vi "OP600ZP_CLUSTER_SOFTS.vi"(10 "MESURES":T1, 11 "EmptyTab":string[][](array[string])) -> (4 "Tab1":string[][](array[string]), 6 "PASS/FAIL":bool[](array[boolean]))   [LabVIEW 2020]
uses:
  VG/PackType.vi
  VG/IS30%.vi
  OP600ZP_VGConf.vi
panel:
  out "VG IS30% ?":bool
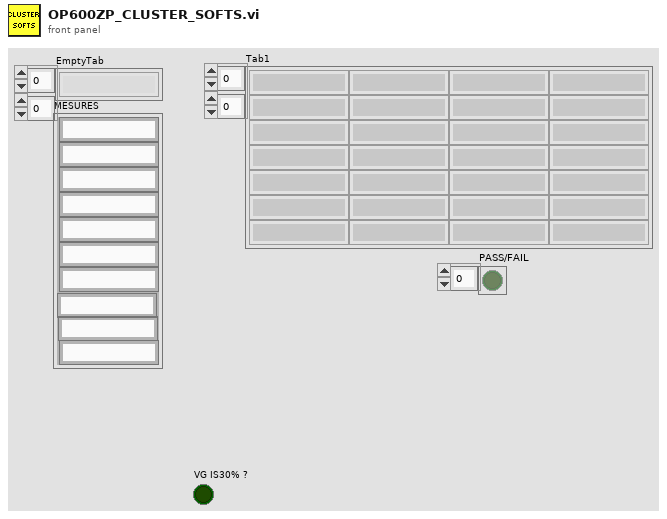
[diagram p1: front panel]
types:
  T1 = cluster{string, string, string, string, string, string, string, string, string, string}
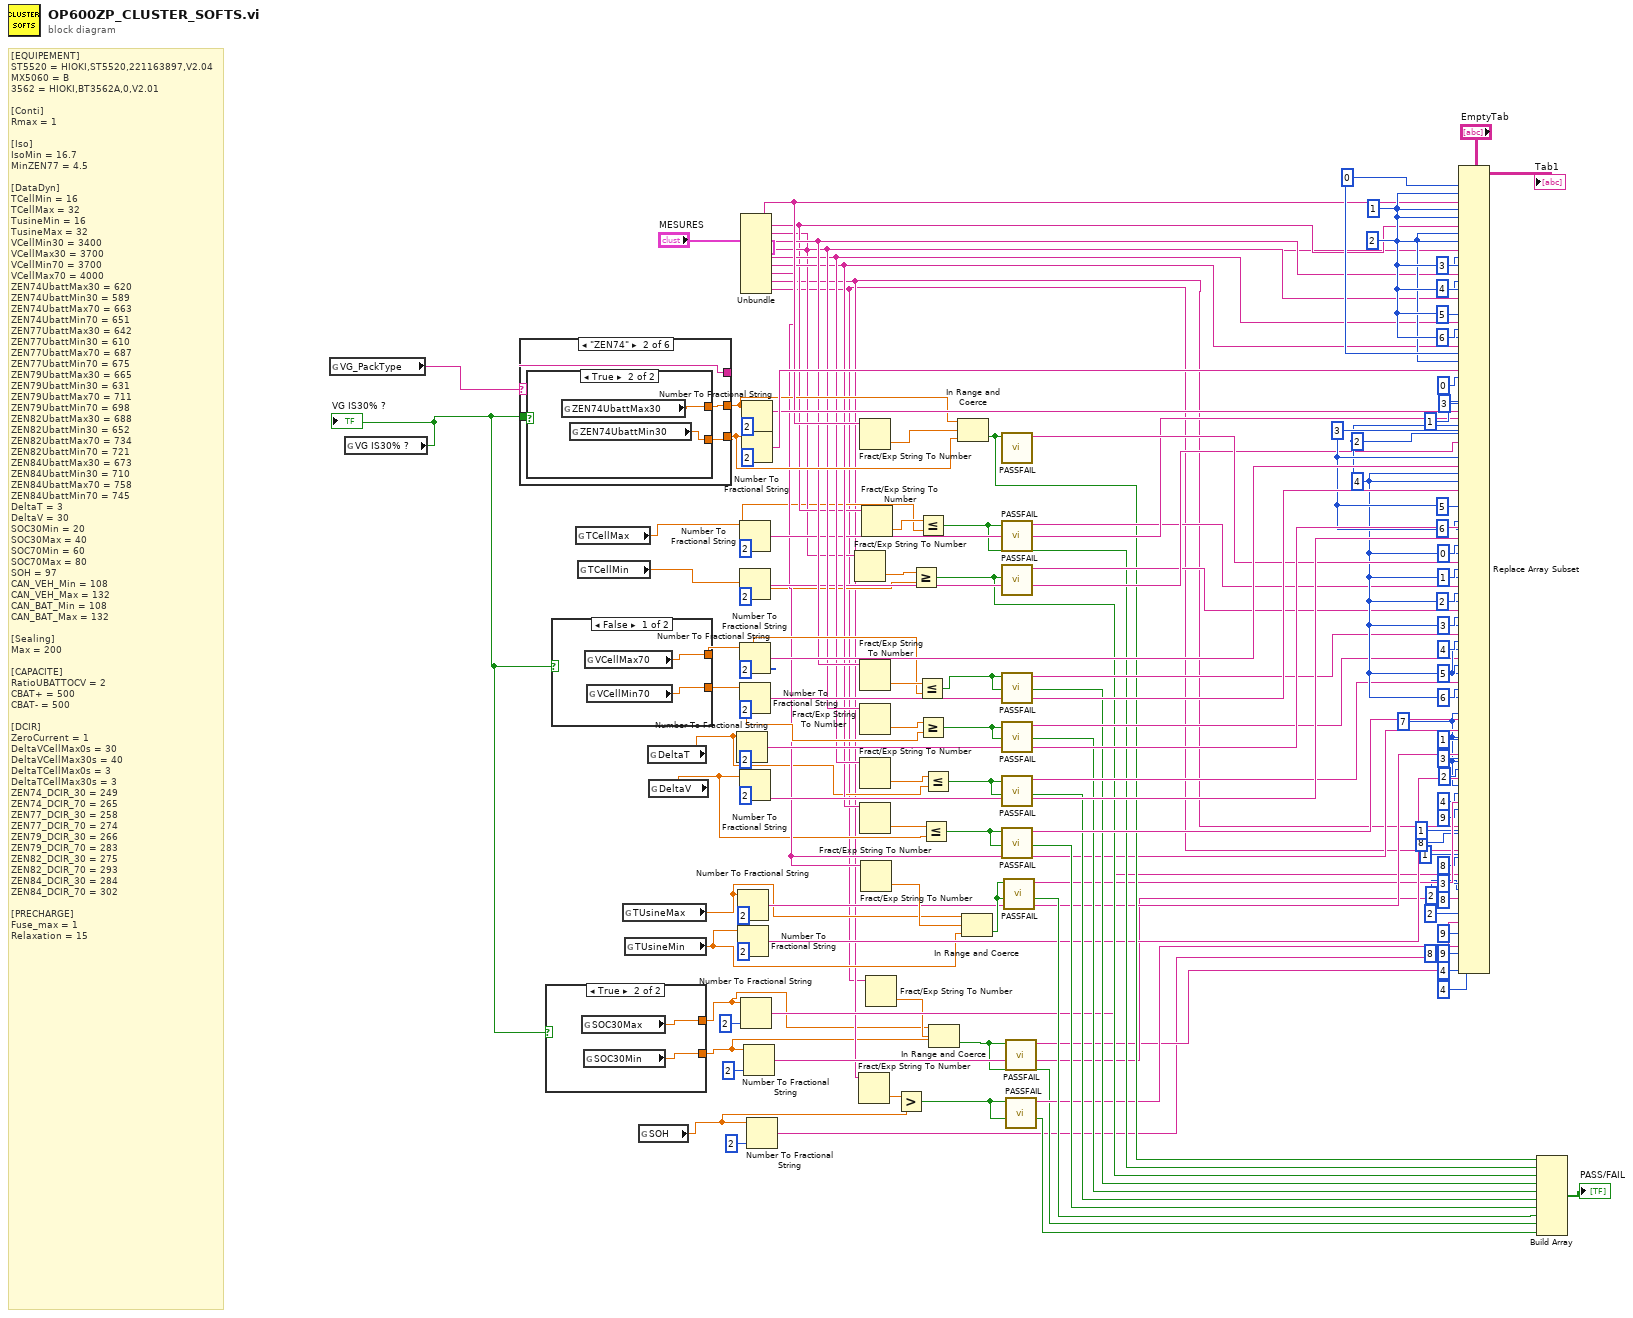
[diagram p0: block diagram]
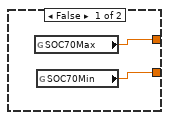
[diagram p2: hidden frame]
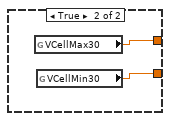
[diagram p3: hidden frame]
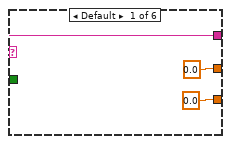
[diagram p4: hidden frame]
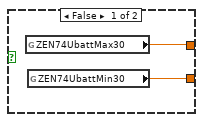
[diagram p5: hidden frame]
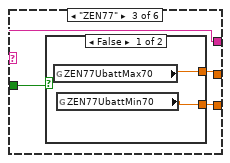
[diagram p6: hidden frame]
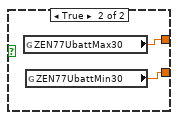
[diagram p7: hidden frame]
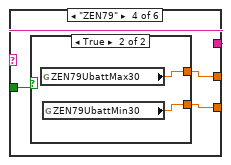
[diagram p8: hidden frame]
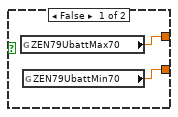
[diagram p9: hidden frame]
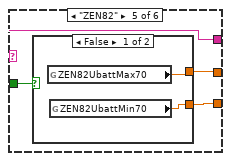
[diagram p10: hidden frame]
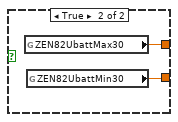
[diagram p11: hidden frame]
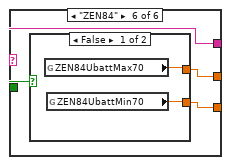
[diagram p12: hidden frame]
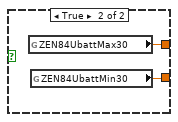
[diagram p13: hidden frame]
diagram:
  w43 = 7 ("indice (ligne)")
  w98 = 2 ("indice désactivé (ligne)")
  w70 = 4 ("indice (ligne)")
  w99 = 3 ("indice désactivé (col)")
  w111 = 2 ("indice désactivé (ligne)")
  w118 = 1 ("indice (col)")
  w121 = 0 ("indice (ligne)")
  # "[EQUIPEMENT]\nST5520 = HIOKI,ST5520,221163897,V2.04\t\nMX5060 = B\n3562 = HIOKI,BT3562A,0,V2.01\n\n[Conti]\nRmax = 1\n\n[Iso]\nIsoMin = 16.7\nMinZEN77 = 4.5\n\n[DataDyn]\nTCellMin = 16\nTCellMax = 32\nTusineMin = 16\nTusineMax = 32\nVCellMin30 = 3400\nVCellMax30 = 3700\nVCellMin70 = 3700\nVCellMax70 = 4000\nZEN74UbattMax30 = 620\nZEN74UbattMin30 = 589\nZEN74UbattMax70 = 663\nZEN74UbattMin70 = 651\nZEN77UbattMax30 = 642\nZEN77UbattMin30 = 610\nZEN77UbattMax70 = 687\nZEN77UbattMin70 = 675\nZEN79UbattMax30 = 665\nZEN79UbattMin30 = 631\nZEN79UbattMax70 = 711\nZEN79UbattMin70 = 698\nZEN82UbattMax30 = 688\nZEN82UbattMin30 = 652\nZEN82UbattMax70 = 734\nZEN82UbattMin70 = 721\nZEN84UbattMax30 = 673\nZEN84UbattMin30 = 710\nZEN84UbattMax70 = 758\nZEN84UbattMin70 = 745\nDeltaT = 3\nDeltaV = 30\nSOC30Min = 20\nSOC30Max = 40\nSOC70Min = 60\nSOC70Max = 80\nSOH = 97\nCAN_VEH_Min = 108\nCAN_VEH_Max = 132\nCAN_BAT_Min = 108\nCAN_BAT_Max = 132\n\n[Sealing]\nMax = 200\n\n[CAPACITE]\nRatioUBATTOCV = 2\nCBAT+ = 500\nCBAT- = 500\n\n[DCIR]\nZeroCurrent = 1\nDeltaVCellMax0s = 30\nDeltaVCellMax30s = 40\nDeltaTCellMax0s = 3\nDeltaTCellMax30s = 3\nZEN74_DCIR_30 = 249\nZEN74_DCIR_70 = 265\nZEN77_DCIR_30 = 258\nZEN77_DCIR_70 = 274\nZEN79_DCIR_30 = 266\nZEN79_DCIR_70 = 283\nZEN82_DCIR_30 = 275\nZEN82_DCIR_70 = 293\nZEN84_DCIR_30 = 284\nZEN84_DCIR_70 = 302\n\n[PRECHARGE]\nFuse_max = 1\nRelaxation = 15"
  n1 = global read "PackType.vi" "VG_PackType"() -> (w37:string)
  n2 = global read "IS30%.vi" "VG IS30% ?"() -> (w28:bool)
  "VG IS30% ?" <- w28
  n3 = case shown="\"ZEN74\"" w37 {
    selector: w37 -> [w129 w130 w138 w146 w154 w162]
    tunnel: [0.0 ("ZEN84UbattMax30") w133 w141 w149 w157 w165] -> w95
    tunnel: [0.0 ("ZEN84UbattMin30") w132 w140 w148 w156 w164] -> w94
    tunnel: w28 -> [_ w131 w139 w147 w155 w163]
    tunnel: [w129 w130 w138 w146 w154 w162] -> _
    frame Default {
    }
    frame "ZEN74" {
      n4 = case shown="True" w131 {
        tunnel: [w135 w137] -> w133
        tunnel: [w134 w136] -> w132
        frame False {
          n5 = global read "OP600ZP_VGConf.vi" "ZEN74UbattMax30"() -> (w135:dbl)
          n6 = global read "OP600ZP_VGConf.vi" "ZEN74UbattMin30"() -> (w134:dbl)
        }
        frame True {
          n7 = global read "OP600ZP_VGConf.vi" "ZEN74UbattMax30"() -> (w137:dbl)
          n8 = global read "OP600ZP_VGConf.vi" "ZEN74UbattMin30"() -> (w136:dbl)
        }
      }
    }
    frame "ZEN77" {
      n9 = case shown="False" w139 {
        tunnel: [w143 w145] -> w141
        tunnel: [w142 w144] -> w140
        frame False {
          n10 = global read "OP600ZP_VGConf.vi" "ZEN77UbattMax70"() -> (w143:dbl)
          n11 = global read "OP600ZP_VGConf.vi" "ZEN77UbattMin70"() -> (w142:dbl)
        }
        frame True {
          n12 = global read "OP600ZP_VGConf.vi" "ZEN77UbattMax30"() -> (w145:dbl)
          n13 = global read "OP600ZP_VGConf.vi" "ZEN77UbattMin30"() -> (w144:dbl)
        }
      }
    }
    frame "ZEN79" {
      n14 = case shown="True" w147 {
        tunnel: [w151 w153] -> w149
        tunnel: [w150 w152] -> w148
        frame False {
          n15 = global read "OP600ZP_VGConf.vi" "ZEN79UbattMax70"() -> (w151:dbl)
          n16 = global read "OP600ZP_VGConf.vi" "ZEN79UbattMin70"() -> (w150:dbl)
        }
        frame True {
          n17 = global read "OP600ZP_VGConf.vi" "ZEN79UbattMax30"() -> (w153:dbl)
          n18 = global read "OP600ZP_VGConf.vi" "ZEN79UbattMin30"() -> (w152:dbl)
        }
      }
    }
    frame "ZEN82" {
      n19 = case shown="False" w155 {
        tunnel: [w159 w161] -> w157
        tunnel: [w158 w160] -> w156
        frame False {
          n20 = global read "OP600ZP_VGConf.vi" "ZEN82UbattMax70"() -> (w159:dbl)
          n21 = global read "OP600ZP_VGConf.vi" "ZEN82UbattMin70"() -> (w158:dbl)
        }
        frame True {
          n22 = global read "OP600ZP_VGConf.vi" "ZEN82UbattMax30"() -> (w161:dbl)
          n23 = global read "OP600ZP_VGConf.vi" "ZEN82UbattMin30"() -> (w160:dbl)
        }
      }
    }
    frame "ZEN84" {
      n24 = case shown="False" w163 {
        tunnel: [w167 w169] -> w165
        tunnel: [w166 w168] -> w164
        frame False {
          n25 = global read "OP600ZP_VGConf.vi" "ZEN84UbattMax70"() -> (w167:dbl)
          n26 = global read "OP600ZP_VGConf.vi" "ZEN84UbattMin70"() -> (w166:dbl)
        }
        frame True {
          n27 = global read "OP600ZP_VGConf.vi" "ZEN84UbattMax30"() -> (w169:dbl)
          n28 = global read "OP600ZP_VGConf.vi" "ZEN84UbattMin30"() -> (w168:dbl)
        }
      }
    }
  }
  n29 = case shown="True" w28 {
    tunnel: [w171 w173] -> w8
    tunnel: [w170 w172] -> w7
    frame False {
      n30 = global read "OP600ZP_VGConf.vi" "SOC70Max"() -> (w171:dbl)
      n31 = global read "OP600ZP_VGConf.vi" "SOC70Min"() -> (w170:dbl)
    }
    frame True {
      n32 = global read "OP600ZP_VGConf.vi" "SOC30Max"() -> (w173:dbl)
      n33 = global read "OP600ZP_VGConf.vi" "SOC30Min"() -> (w172:dbl)
    }
  }
  n34 = case shown="False" w28 {
    tunnel: [w175 w177] -> w92
    tunnel: [w174 w176] -> w88
    frame False {
      n35 = global read "OP600ZP_VGConf.vi" "VCellMax70"() -> (w175:dbl)
      n36 = global read "OP600ZP_VGConf.vi" "VCellMin70"() -> (w174:dbl)
    }
    frame True {
      n37 = global read "OP600ZP_VGConf.vi" "VCellMax30"() -> (w177:dbl)
      n38 = global read "OP600ZP_VGConf.vi" "VCellMin30"() -> (w176:dbl)
    }
  }
  n39 = global read "OP600ZP_VGConf.vi" "TCellMax"() -> (w36:dbl)
  n40 = global read "OP600ZP_VGConf.vi" "TCellMin"() -> (w35:dbl)
  n41 = global read "OP600ZP_VGConf.vi" "TUsineMax"() -> (w32:dbl)
  n42 = global read "OP600ZP_VGConf.vi" "TUsineMin"() -> (w31:dbl)
  n43 = global read "OP600ZP_VGConf.vi" "SOH"() -> (w16:dbl)
  n44 = global read "OP600ZP_VGConf.vi" "DeltaT"() -> (w34:dbl)
  n45 = global read "OP600ZP_VGConf.vi" "DeltaV"() -> (w33:dbl)
  n46 = Number To Fractional String(number=w34, precision (6)=i16 2 ("précision (6)")) -> (F-format string=w103:string)  [unwired: 2 in]
  n47 = Number To Fractional String(number=w32, precision (6)=i16 2 ("précision (6)")) -> (F-format string=w48:string)  [unwired: 2 in]
  n48 = Number To Fractional String(number=w31, precision (6)=i16 2 ("précision (6)")) -> (F-format string=w47:string)  [unwired: 2 in]
  n49 = Number To Fractional String(number=w36, precision (6)=i16 2 ("précision (6)")) -> (F-format string=w73:string)  [unwired: 2 in]
  n50 = Number To Fractional String(number=w35, precision (6)=i16 2 ("précision (6)")) -> (F-format string=w74:string)  [unwired: 2 in]
  n51 = Number To Fractional String(number=w92, precision (6)=i16 2 ("précision (6)")) -> (F-format string=w108:string)  [unwired: 2 in]
  n52 = Number To Fractional String(number=w88, precision (6)=i16 2 ("précision (6)")) -> (F-format string=w106:string)  [unwired: 2 in]
  n53 = Number To Fractional String(number=w33, precision (6)=i16 2 ("précision (6)")) -> (F-format string=w102:string)  [unwired: 2 in]
  n54 = Unbundle("MESURES") -> (w97:string, w63:string, w62:string, w91:string, w89:string, w86:string, w85:string, w52:string, w15:string, w10:string)
  n55 = Number To Fractional String(number=w8, precision (6)=i16 2 ("précision (6)")) -> (F-format string=w25:string)  [unwired: 2 in]
  n56 = Number To Fractional String(number=w95, precision (6)=i16 2 ("précision (6)")) -> (F-format string=w119:string)  [unwired: 2 in]
  n57 = Number To Fractional String(number=w94, precision (6)=i16 2 ("précision (6)")) -> (F-format string=w120:string)  [unwired: 2 in]
  n58 = Number To Fractional String(number=w7, precision (6)=i16 2 ("précision (6)")) -> (F-format string=w24:string)  [unwired: 2 in]
  n59 = Number To Fractional String(number=w16, precision (6)=i16 2 ("précision (6)")) -> (F-format string=w1:string)  [unwired: 2 in]
  n60 = Fract/Exp String To Number(string=w62) -> (number=w83:dbl)  [unwired: 3 in, 1 out]
  n61 = Fract/Exp String To Number(string=w15) -> (number=w14:dbl)  [unwired: 3 in, 1 out]
  n62 = Fract/Exp String To Number(string=w97) -> (number=w96:dbl)  [unwired: 3 in, 1 out]
  n63 = Fract/Exp String To Number(string=w91) -> (number=w93:dbl)  [unwired: 3 in, 1 out]
  n64 = Fract/Exp String To Number(string=w89) -> (number=w90:dbl)  [unwired: 3 in, 1 out]
  n65 = Fract/Exp String To Number(string=w86) -> (number=w61:dbl)  [unwired: 3 in, 1 out]
  n66 = Fract/Exp String To Number(string=w85) -> (number=w87:dbl)  [unwired: 3 in, 1 out]
  n67 = Fract/Exp String To Number(string=w52) -> (number=w50:dbl)  [unwired: 3 in, 1 out]
  n68 = Fract/Exp String To Number(string=w63) -> (number=w84:dbl)  [unwired: 3 in, 1 out]
  n69 = Fract/Exp String To Number(string=w10) -> (number=w9:dbl)  [unwired: 3 in, 1 out]
  n70 = Greater?(x=w14, y=w16) -> (0:w6:bool)
  n71 = Greater Or Equal?(x=w83, y=w35) -> (x >= y?=w58:bool)
  n72 = Less Or Equal?(x=w93, y=w92) -> (x <= y?=w57:bool)
  n73 = Less Or Equal?(x=w84, y=w36) -> (x <= y?=w59:bool)
  n74 = Greater Or Equal?(x=w90, y=w88) -> (x >= y?=w56:bool)
  n75 = Less Or Equal?(x=w87, y=w33) -> (x <= y?=w54:bool)
  n76 = Less Or Equal?(x=w61, y=w34) -> (x <= y?=w55:bool)
  n77 = In Range and Coerce(upper limit=w8, x=w9, lower limit=w7) -> (In Range?=w5:bool)  [unwired: 1 out]
  n78 = In Range and Coerce(upper limit=w95, x=w96, lower limit=w94) -> (In Range?=w60:bool)  [unwired: 1 out]
  n79 = In Range and Coerce(upper limit=w32, x=w50, lower limit=w31) -> (In Range?=w49:bool)  [unwired: 1 out]
  n80 = call <userlib>:"PASSFAIL.vi"("E"=w60) -> ("S"=w80:string)  [unwired: 10 in]
  n81 = call <userlib>:"PASSFAIL.vi"("E"=w59) -> ("S"=w69:string)  [unwired: 10 in]
  n82 = call <userlib>:"PASSFAIL.vi"("E"=w58) -> ("S"=w68:string)  [unwired: 10 in]
  n83 = call <userlib>:"PASSFAIL.vi"("E"=w57) -> ("S"=w67:string)  [unwired: 10 in]
  n84 = call <userlib>:"PASSFAIL.vi"("E"=w56) -> ("S"=w66:string)  [unwired: 10 in]
  n85 = call <userlib>:"PASSFAIL.vi"("E"=w55) -> ("S"=w65:string)  [unwired: 10 in]
  n86 = call <userlib>:"PASSFAIL.vi"("E"=w54) -> ("S"=w64:string)  [unwired: 10 in]
  n87 = call <userlib>:"PASSFAIL.vi"("E"=w49) -> ("S"=w44:string)  [unwired: 10 in]
  n88 = call <userlib>:"PASSFAIL.vi"("E"=w5) -> ("S"=w4:string)  [unwired: 10 in]
  n89 = call <userlib>:"PASSFAIL.vi"("E"=w6) -> ("S"=w13:string)  [unwired: 10 in]
  n90 = Replace Array Subset(array="EmptyTab", new element #1=w97, index (row) #1=w121, index (col) #1=w118, new element #2=w63, index (row) #2=w118, index (col) #2=w118, new element #3=w62, index (row) #3=w111, index (col) #3=w118, new element #4=w91, index (row) #4=3 ("indice désactivé (ligne)"), index (col) #4=w118, new element #5=w89, index (row) #5=4 ("indice désactivé (ligne)"), index (col) #5=w118, new element #6=w86, index (row) #6=5 ("indice désactivé (ligne)"), index (col) #6=w118, new element #7=w85, index (row) #7=6 ("indice désactivé (ligne)"), index (col) #7=w118, new element #8=w120, index (row) #8=w121, index (col) #8=w111, new element #9=w119, index (row) #9=0 ("indice (ligne)"), index (col) #9=3 ("indice désactivé (col)"), new element #10=w73, index (row) #10=1 ("indice désactivé (ligne)"), index (col) #10=w99, new element #11=w74, index (row) #11=w98, index (col) #11=w98, new element #12=w108, index (row) #12=w99, index (col) #12=w99, new element #13=w106, index (row) #13=w70, index (col) #13=w98, new element #14=w103, index (row) #14=5 ("indice (ligne)"), index (col) #14=w99, new element #15=w102, index (row) #15=6 ("indice désactivé (ligne)"), index (col) #15=w99, new element #16=w80, index (row) #16=0 ("indice (ligne)"), index (col) #16=w70, new element #17=w69, index (row) #17=1 ("indice (ligne)"), index (col) #17=w70, new element #18=w68, index (row) #18=2 ("indice (ligne)"), index (col) #18=w70, new element #19=w67, index (row) #19=3 ("indice (ligne)"), index (col) #19=w70, new element #20=w66, index (row) #20=4 ("indice (ligne)"), index (col) #20=w70, new element #21=w65, index (row) #21=5 ("indice (ligne)"), index (col) #21=w70, new element #22=w64, index (row) #22=6 ("indice (ligne)"), index (col) #22=w70, new element #23=w52, index (row) #23=w43, index (col) #23=1 ("indice désactivé (col)"), new element #24=w48, index (row) #24=w43, index (col) #24=3 ("indice désactivé (col)"), new element #25=w47, index (row) #25=w43, index (col) #25=2 ("indice désactivé (col)"), new element #26=w44, index (row) #26=w43, index (col) #26=4 ("indice désactivé (col)"), new element #27=w15, index (row) #27=9 ("indice (ligne)"), index (col) #27=1 ("indice désactivé (col)"), new element #28=w10, index (row) #28=8 ("indice (ligne)"), index (col) #28=1 ("indice désactivé (col)"), new element #29=w25, index (row) #29=8 ("indice (ligne)"), index (col) #29=3 ("indice désactivé (col)"), new element #30=w24, index (row) #30=8 ("indice (ligne)"), index (col) #30=2 ("indice désactivé (col)"), new element #31=w1, index (row) #31=9 ("indice (ligne)"), index (col) #31=2 ("indice désactivé (col)"), new element #32=w13, index (row) #32=9 ("indice (ligne)"), index (col) #32=4 ("indice désactivé (col)"), new element #33=w4, index (row) #33=8 ("indice (ligne)"), index (col) #33=4 ("indice désactivé (col)")) -> (→"Tab1":string[][])
  n91 = Build Array(w60, w59, w58, w57, w56, w55, w54, w49, w5, w6) -> (→"PASS/FAIL":bool[])
